vi "Teleop_System_Calc_Drive_Mode.vi"(8 "Traj Rev Follow Orient":bool, 9 "Traj Rev Same Orient":bool, 10 "Traj Fwd Follow Orient":bool, 11 "Traj Fwd Same Orient":bool) -> (2 "Dirve Mode Changed":bool, 3 "Drive Mode":i32)   [LabVIEW 2019]
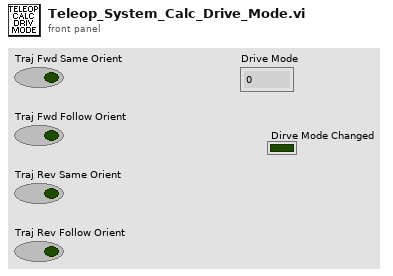
[diagram p1: front panel]
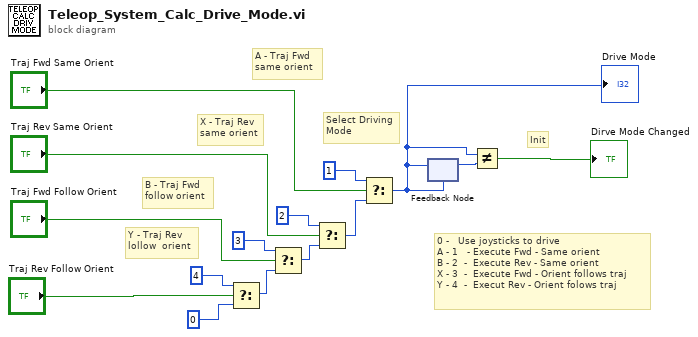
[diagram p0: block diagram]
diagram:
  # "0 -   Use joysticks to drive\nA - 1   - Execute Fwd - Same orient\nB - 2  -  Execute Rev - Same orient\nX - 3  -  Execute Fwd - Orient follows traj\nY - 4  -  Execut Rev - Orient folows traj"
  # "Init"
  # "Y - Traj Rev \nlollow  orient"
  # "B - Traj Fwd \nfollow orient"
  # "X - Traj Rev\nsame orient"
  # "A - Traj Fwd \nsame orient"
  # "Select Driving\nMode"
  n1 = Select(t=4, s="Traj Rev Follow Orient", f=0) -> (s? t:f=w12:i32)
  n2 = Select(t=3, s="Traj Fwd Follow Orient", f=w12) -> (s? t:f=w11:i32)
  n3 = Select(t=2, s="Traj Rev Same Orient", f=w11) -> (s? t:f=w7:i32)
  n4 = Select(t=1, s="Traj Fwd Same Orient", f=w7) -> (s? t:f=w4:i32)
  "Drive Mode" <- w4
  n5 = feedback #1(w4) -> (w3:i32)
  n6 = feedback-in #1(w4) -> ()
  n7 = Not Equal?(x=w4, y=w3) -> (x != y?=→"Dirve Mode Changed":bool)
